vi "ConvertVoltageToPWM.vi"(1 "Numérique en entrée":dbl) -> (0 "Numérique en sortie":u8)   [LabVIEW 2021]
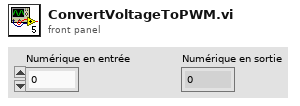
[diagram p1: front panel]
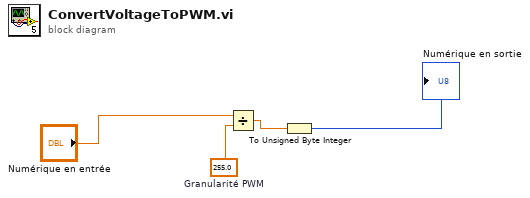
[diagram p0: block diagram]
diagram:
  w2 = 255.0  # Granularité PWM
  n1 = Divide(x="Numérique en entrée", y=w2) -> (x/y=w3:dbl)
  n2 = To Unsigned Byte Integer(number=w3) -> (unsigned 8bit integer=→"Numérique en sortie":u8)
